vi "RT DC SERVO.vi"() -> ()   [LabVIEW 2015]
uses:
  <vilib>/Utility/error.llb/DialogType.ctl
  SAMPLE DO LED/Control 3.ctl
  <vilib>/FPGAPlugInAG/myRIO-1900/niLvFpga_Open_myRIO-1900.vi
  <vilib>/rvi/interface/common/dynamic/niFpgaDynamicAddResources.vi
  <vilib>/Utility/error.llb/Error Cluster From Error Code.vi
  <vilib>/rvi/errors/niLvFpgaAdjustHostInterfaceError.vi
  <vilib>/FPGAPlugInAG/Dynamic/niLvFpga_Close_Dynamic.vi
  <vilib>/rvi/interface/nirviOpenFPGA/nirviOpenFPGA.xnode
  FPGA Bitfiles/DCSERVO_FPGATarget_FPGADCSERVO_HoNCdCg9UOQ.lvbitx
  FPGA DC SERVO.vi
  <vilib>/rvi/interface/nirviReadWriteControl/nirviReadWriteControl.xnode
  <vilib>/rvi/interface/nirviCloseFPGA/nirviCloseFPGA.xnode
  NiFpgaLv.dll
  <vilib>/rvi/interface/Simulation/niFpgaSimulationCallBeginRW.vi
panel:
  out "Sudut":dbl(knob) min=0.0 max=180.0 step=1.0 scale=0.0..180.0
  in  "stop":bool
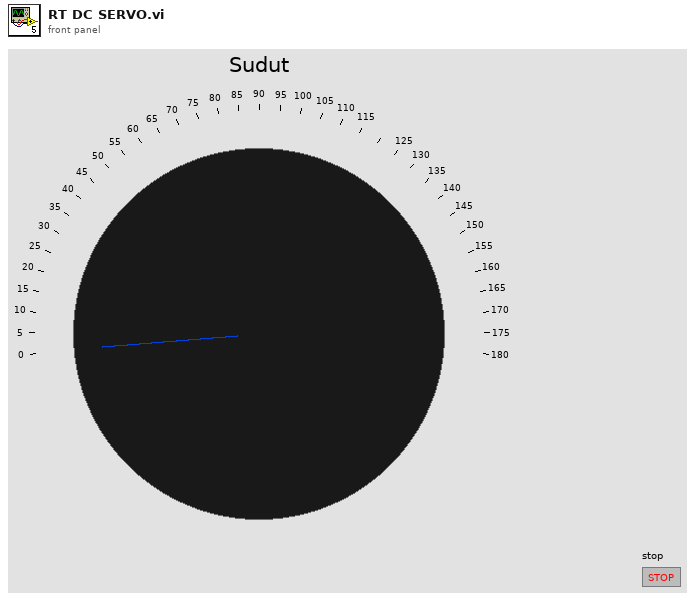
[diagram p1: front panel]
types:
  T1 = typedef "Control 3.ctl" = enum16{"Start", "0", "0 2", "30", "30 2", "60", "90", "delay1", "delay2", "delay3", "delay4", "delay5", "return", "stop"}
  T2 = typedef "DialogType.ctl" = u16
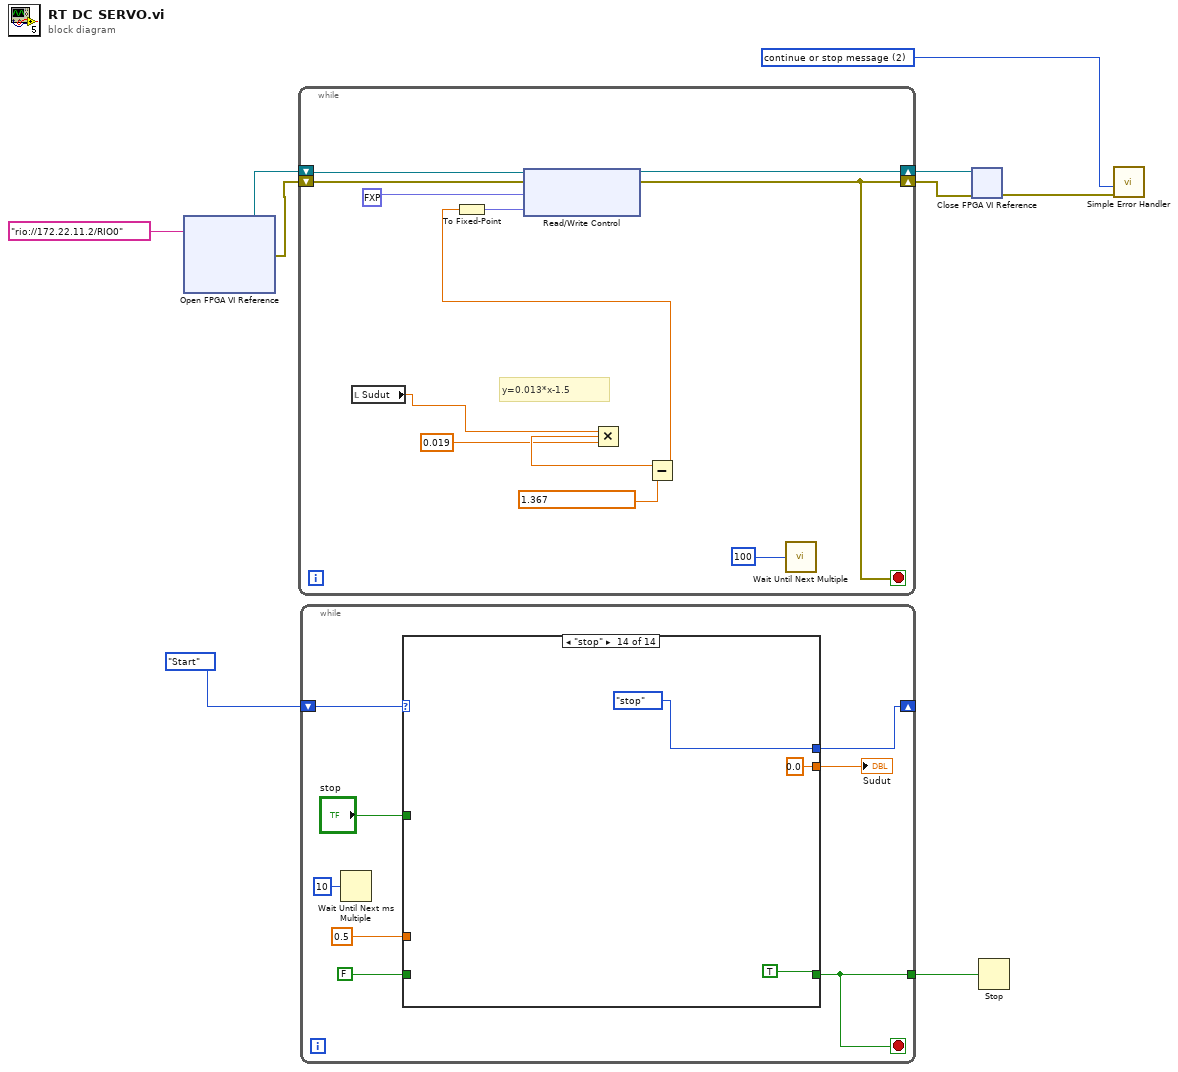
[diagram p0: block diagram]
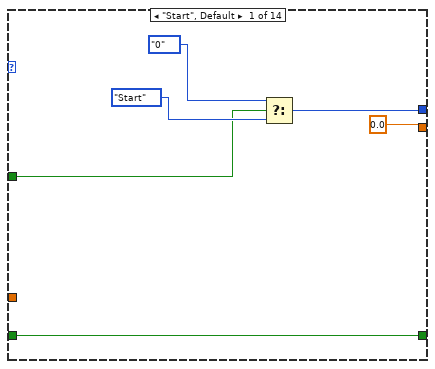
[diagram p2: hidden frame]
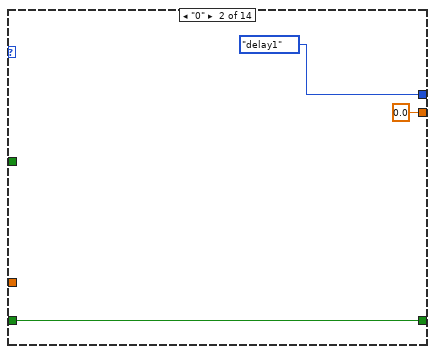
[diagram p3: hidden frame]
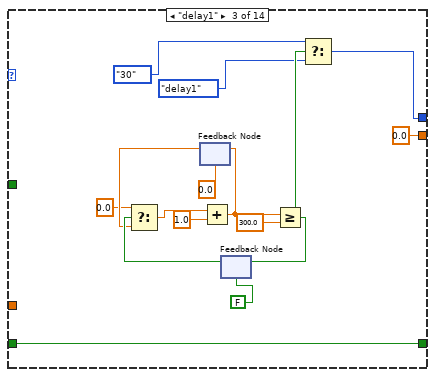
[diagram p4: hidden frame]
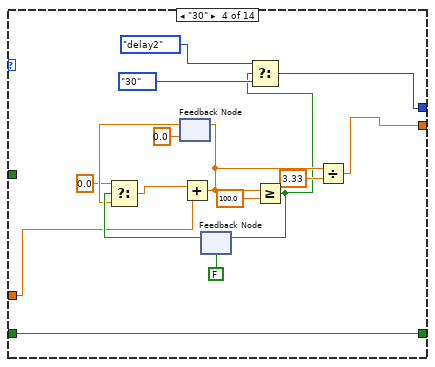
[diagram p5: hidden frame]
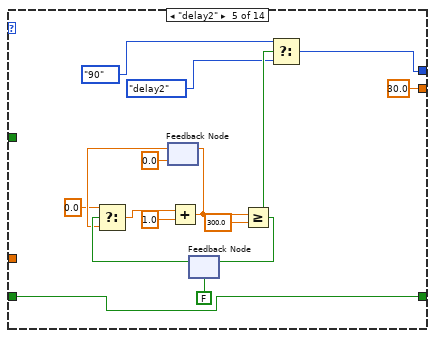
[diagram p6: hidden frame]
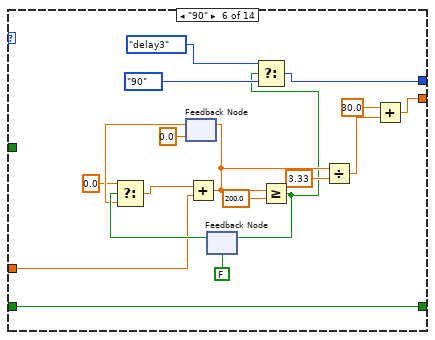
[diagram p7: hidden frame]
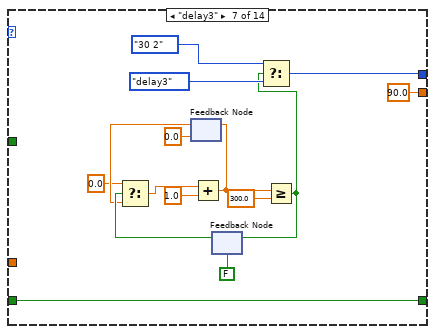
[diagram p8: hidden frame]
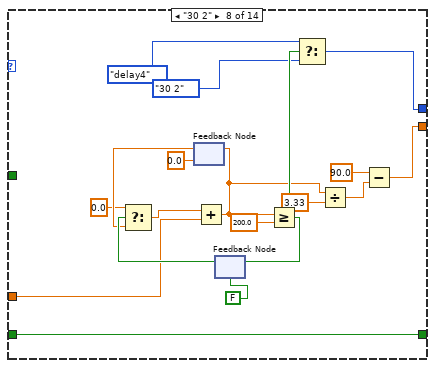
[diagram p9: hidden frame]
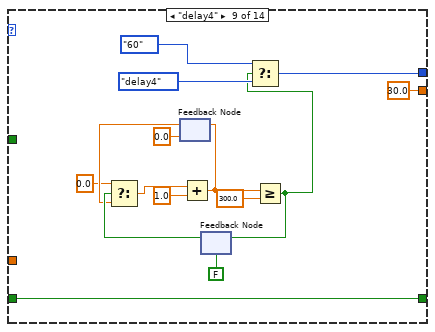
[diagram p10: hidden frame]
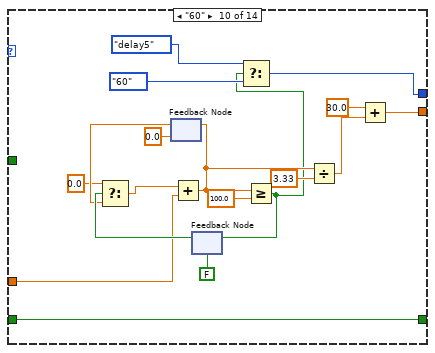
[diagram p11: hidden frame]
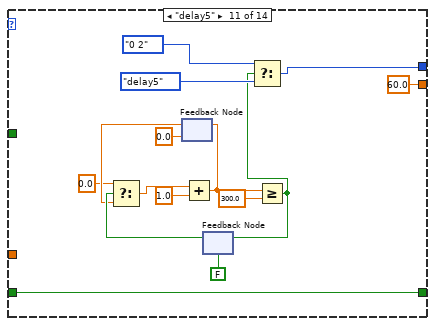
[diagram p12: hidden frame]
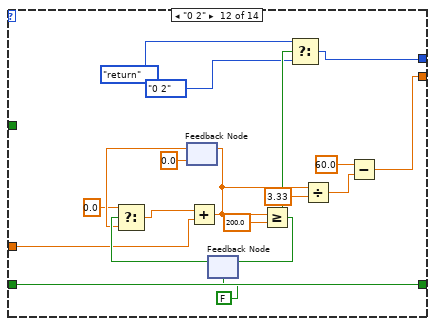
[diagram p13: hidden frame]
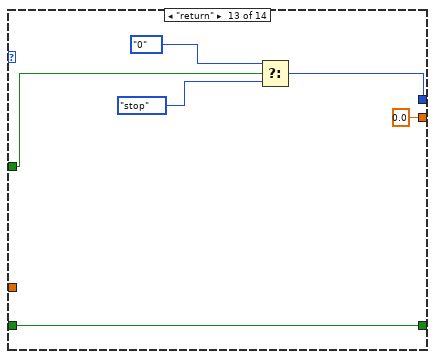
[diagram p14: hidden frame]
diagram:
  w6 = T2 2 items=["no dialog", "OK message", "continue or stop message", "OK message + warnings", "continue/stop + warnings"] ("type of dialog (OK msg:1)")
  n1 = xnode "Open FPGA VI Reference"("resource name"=tag "rio://172.22.11.2/RIO0") -> ("FPGA VI Reference Out"=w4:refnum<k20>, "error out"=w3:errorcluster)  [unwired: 1 in]
  n2 = while {
    shift-right: [w18] -> w9
    shift-left: w4 -> [w21]
    shift-right: [w17] -> w8
    shift-left: w3 -> [w20]
    stop <- w17 stop-if-true
    # "y=0.013*x-1.5"
    n3 = local read "Sudut"() -> (w10:dbl)
    n4 = Multiply(x=w10, y=0.019) -> (x*y=w15:dbl)
    n5 = Subtract(x=w15, y=1.367) -> (x-y=w13:dbl)
    n6 = To Fixed-Point(number=w13) -> (fixed-point=w12:fxp<+/-,32,16>)  [unwired: 1 in]
    n7 = xnode "Read/Write Control"("FPGA VI Reference In"=w21, "error in"=w20, "servo_0_ccw offset"=fxp<+/-,32,4> 0.0, "servo_0_ccw angle"=w12) -> ("FPGA VI Reference Out"=w18:refnum<k20>, "error out"=w17:errorcluster)
    n8 = call "Wait Until Next Multiple"("Count(mSec)"=u32 100) -> ()  [unwired: 1 out]
  }
  n9 = while {
    shift-right: [w22] -> _
    shift-left: Control_3."Start" -> [w27]
    tunnel: [w23] -> w2
    stop <- w23 stop-if-true
    n10 = Wait Until Next ms Multiple(millisecond multiple=u32 10) -> ()  [unwired: 1 out]
    n11 = case shown="\"stop\"" w27 {
      tunnel: [0.0 0.0 0.0 w54 30.0 w86 90.0 w123 30.0 w155 60.0 w185 0.0 0.0] -> w28
      tunnel: "stop" -> [w31 _ _ _ _ _ _ _ _ _ _ _ w202 _]
      tunnel: 0.5 -> [_ _ _ w58 _ w87 _ w125 _ w159 _ w190 _ _]
      tunnel: FALSE -> [w30 w36 w39 w55 w72 w85 w103 w119 w136 w153 w169 w192 w206 _]
      tunnel: [w30 w36 w39 w55 w72 w85 w103 w119 w136 w153 w169 w192 w206 TRUE] -> w23
      tunnel: [w32 Control_3."delay1" w44 w57 w82 w89 w106 w127 w138 w152 w171 w193 w203 Control_3."stop"] -> w22
      frame "Start", Default {
        n12 = Select(t=Control_3."0", s=w31, f=Control_3."Start") -> (s? t:f=w32:T1)
      }
      frame "0" {
      }
      frame "delay1" {
        n13 = feedback #1(0.0) -> (w50:dbl)
        n14 = feedback #2(FALSE) -> (w51:bool)
        n15 = Select(t=0.0, s=w51, f=w50) -> (s? t:f=w53:dbl)
        n16 = Add(x=w53, y=1.0) -> (x+y=w48:dbl)
        n17 = feedback-in #1(w48) -> ()
        n18 = Greater Or Equal?(x=w48, y=300.0) -> (x >= y?=w52:bool)
        n19 = feedback-in #2(w52) -> ()
        n20 = Select(t=Control_3."30", s=w52, f=Control_3."delay1") -> (s? t:f=w44:T1)
      }
      frame "30" {
        n21 = feedback #3(0.0) -> (w64:dbl)
        n22 = feedback #4(FALSE) -> (w66:bool)
        n23 = Select(t=0.0, s=w66, f=w64) -> (s? t:f=w67:dbl)
        n24 = Add(x=w67, y=w58) -> (x+y=w59:dbl)
        n25 = feedback-in #3(w59) -> ()
        n26 = Greater Or Equal?(x=w59, y=100.0) -> (x >= y?=w56:bool)
        n27 = feedback-in #4(w56) -> ()
        n28 = Select(t=Control_3."delay2", s=w56, f=Control_3."30") -> (s? t:f=w57:T1)
        n29 = Divide(x=w59, y=3.33) -> (x/y=w54:dbl)
      }
      frame "delay2" {
        n30 = feedback #5(0.0) -> (w78:dbl)
        n31 = feedback #6(FALSE) -> (w80:bool)
        n32 = Select(t=0.0, s=w80, f=w78) -> (s? t:f=w83:dbl)
        n33 = Add(x=w83, y=1.0) -> (x+y=w76:dbl)
        n34 = feedback-in #5(w76) -> ()
        n35 = Greater Or Equal?(x=w76, y=300.0) -> (x >= y?=w81:bool)
        n36 = feedback-in #6(w81) -> ()
        n37 = Select(t=Control_3."90", s=w81, f=Control_3."delay2") -> (s? t:f=w82:T1)
      }
      frame "90" {
        n38 = feedback #7(0.0) -> (w97:dbl)
        n39 = feedback #8(FALSE) -> (w99:bool)
        n40 = Select(t=0.0, s=w99, f=w97) -> (s? t:f=w100:dbl)
        n41 = Add(x=w100, y=w87) -> (x+y=w92:dbl)
        n42 = feedback-in #7(w92) -> ()
        n43 = Greater Or Equal?(x=w92, y=200.0) -> (x >= y?=w88:bool)
        n44 = feedback-in #8(w88) -> ()
        n45 = Select(t=Control_3."delay3", s=w88, f=Control_3."90") -> (s? t:f=w89:T1)
        n46 = Divide(x=w92, y=3.33) -> (x/y=w91:dbl)
        n47 = Add(x=30.0, y=w91) -> (x+y=w86:dbl)
      }
      frame "delay3" {
        n48 = feedback #9(0.0) -> (w111:dbl)
        n49 = feedback #10(FALSE) -> (w113:bool)
        n50 = Select(t=0.0, s=w113, f=w111) -> (s? t:f=w114:dbl)
        n51 = Add(x=w114, y=1.0) -> (x+y=w107:dbl)
        n52 = feedback-in #9(w107) -> ()
        n53 = Greater Or Equal?(x=w107, y=300.0) -> (x >= y?=w105:bool)
        n54 = feedback-in #10(w105) -> ()
        n55 = Select(t=Control_3."30 2", s=w105, f=Control_3."delay3") -> (s? t:f=w106:T1)
      }
      frame "30 2" {
        n56 = feedback #11(0.0) -> (w132:dbl)
        n57 = feedback #12(FALSE) -> (w133:bool)
        n58 = Select(t=0.0, s=w133, f=w132) -> (s? t:f=w135:dbl)
        n59 = Add(x=w135, y=w125) -> (x+y=w120:dbl)
        n60 = feedback-in #11(w120) -> ()
        n61 = Greater Or Equal?(x=w120, y=200.0) -> (x >= y?=w134:bool)
        n62 = feedback-in #12(w134) -> ()
        n63 = Select(t=Control_3."delay4", s=w134, f=Control_3."30 2") -> (s? t:f=w127:T1)
        n64 = Divide(x=w120, y=3.33) -> (x/y=w124:dbl)
        n65 = Subtract(x=90.0, y=w124) -> (x-y=w123:dbl)
      }
      frame "delay4" {
        n66 = feedback #13(0.0) -> (w144:dbl)
        n67 = feedback #14(FALSE) -> (w146:bool)
        n68 = Select(t=0.0, s=w146, f=w144) -> (s? t:f=w147:dbl)
        n69 = Add(x=w147, y=1.0) -> (x+y=w140:dbl)
        n70 = feedback-in #13(w140) -> ()
        n71 = Greater Or Equal?(x=w140, y=300.0) -> (x >= y?=w137:bool)
        n72 = feedback-in #14(w137) -> ()
        n73 = Select(t=Control_3."60", s=w137, f=Control_3."delay4") -> (s? t:f=w138:T1)
      }
      frame "60" {
        n74 = feedback #15(0.0) -> (w163:dbl)
        n75 = feedback #16(FALSE) -> (w165:bool)
        n76 = Select(t=0.0, s=w165, f=w163) -> (s? t:f=w166:dbl)
        n77 = Add(x=w166, y=w159) -> (x+y=w157:dbl)
        n78 = feedback-in #15(w157) -> ()
        n79 = Greater Or Equal?(x=w157, y=100.0) -> (x >= y?=w151:bool)
        n80 = feedback-in #16(w151) -> ()
        n81 = Select(t=Control_3."delay5", s=w151, f=Control_3."60") -> (s? t:f=w152:T1)
        n82 = Divide(x=w157, y=3.33) -> (x/y=w156:dbl)
        n83 = Add(x=30.0, y=w156) -> (x+y=w155:dbl)
      }
      frame "delay5" {
        n84 = feedback #17(0.0) -> (w177:dbl)
        n85 = feedback #18(FALSE) -> (w179:bool)
        n86 = Select(t=0.0, s=w179, f=w177) -> (s? t:f=w180:dbl)
        n87 = Add(x=w180, y=1.0) -> (x+y=w173:dbl)
        n88 = feedback-in #17(w173) -> ()
        n89 = Greater Or Equal?(x=w173, y=300.0) -> (x >= y?=w170:bool)
        n90 = feedback-in #18(w170) -> ()
        n91 = Select(t=Control_3."0 2", s=w170, f=Control_3."delay5") -> (s? t:f=w171:T1)
      }
      frame "0 2" {
        n92 = feedback #19(0.0) -> (w198:dbl)
        n93 = feedback #20(FALSE) -> (w199:bool)
        n94 = Select(t=0.0, s=w199, f=w198) -> (s? t:f=w201:dbl)
        n95 = Add(x=w201, y=w190) -> (x+y=w189:dbl)
        n96 = feedback-in #19(w189) -> ()
        n97 = Greater Or Equal?(x=w189, y=200.0) -> (x >= y?=w200:bool)
        n98 = feedback-in #20(w200) -> ()
        n99 = Select(t=Control_3."return", s=w200, f=Control_3."0 2") -> (s? t:f=w193:T1)
        n100 = Divide(x=w189, y=3.33) -> (x/y=w187:dbl)
        n101 = Subtract(x=60.0, y=w187) -> (x-y=w185:dbl)
      }
      frame "return" {
        n102 = Select(t=Control_3."0", s=w202, f=Control_3."stop") -> (s? t:f=w203:T1)
      }
      frame "stop" {
      }
    }
    "Sudut" <- w28
  }
  n103 = xnode "Close FPGA VI Reference"("FPGA VI Reference In"=w9, "error in"=w8) -> ("error out"=w7:errorcluster)
  n104 = Stop(stop? (T)=w2) -> ()
  n105 = call <vilib>:"Simple Error Handler.vi"("type of dialog (OK msg:1)"=w6, "error in (no error)"=w7) -> ()  [unwired: 3 in, 5 out]
